vi "LocalQueue_Test No Connection Errors.vi"(8 "error in (no error)":errorcluster) -> (0 "error out":errorcluster)   [LabVIEW 2013]
uses:
  <vilib>/addons/_JKI Toolkits/Caraya/classes/Assert/Assert Equal Value_Variant.vi
  <vilib>/LabVIEW Open Source Project/Connection/Connection/Connection.lvclass
  <vilib>/addons/_JKI Toolkits/Caraya/classes/Test/Test.lvclass
  <vilib>/addons/_JKI Toolkits/Caraya/classes/Assert/Assert.lvclass
  source/MQTT_LocalQueue/Connection/LocalQueueConnection.lvclass
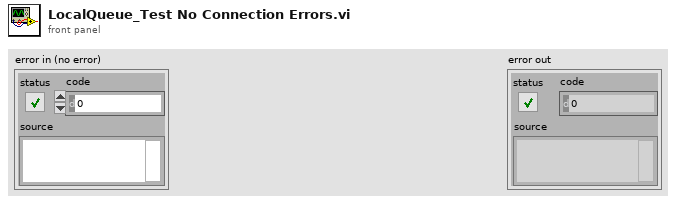
[diagram p1: front panel]
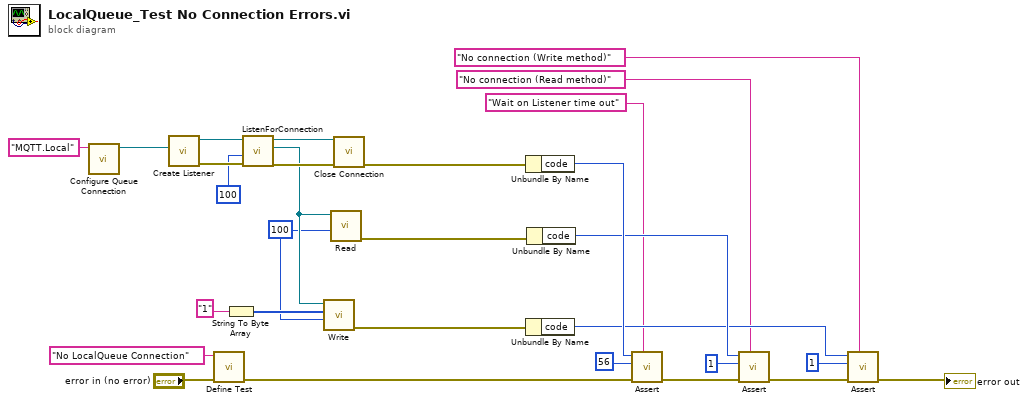
[diagram p0: block diagram]
diagram:
  w3 = 100 ("bytes to read")
  n1 = call "Configure Queue Connection.vi"("Queue Name"="MQTT.Local") -> ("LocalQueueConnection"=w2:refnum<class "LocalQueueConnection.lvclass">)  [unwired: 9 in, 1 out]
  n2 = call <vilib>:"Create Listener.vi"("Connection Configuration"=w2) -> ("error out"=w26:errorcluster, "Listener"=w29:refnum<class "LocalQueueConnection.lvclass">)  [unwired: 9 in]
  n3 = call <vilib>:"Define Test.vi"("error in (no error)"="error in (no error)", "Label (VI Title)"="No LocalQueue Connection") -> ("error out"=w17:errorcluster)  [unwired: 9 in]
  n4 = String To Byte Array(string="1" ("data in")) -> (unsigned byte array=w24:u8[])
  n5 = call <vilib>:"ListenForConnection.vi"("error in (no error)"=w26, "timeout (2000 ms)"=100 ("timeout ms (wait forever: -1)"), "Listener"=w29) -> ("error out"=w27:errorcluster, "Connection"=w22:refnum<class "Connection.lvclass">, "Listener out"=w28:refnum<class "LocalQueueConnection.lvclass">)  [unwired: 5 in, 1 out]
  n6 = call <vilib>:"Write.vi"("timeout (2000 ms)"=w3, "Bytes"=w24, "Connection in"=w22) -> ("error out"=w20:errorcluster)  [unwired: 7 in, 1 out]
  n7 = call <vilib>:"Read.vi"("timeout (2000 ms)"=w3, "TCPConnection in"=w22) -> ("error out"=w19:errorcluster)  [unwired: 5 in, 4 out]
  n8 = call <vilib>:"Close Connection.vi"("error in (no error)"=w27, "Connection in"=w28) -> ("error out"=w21:errorcluster)  [unwired: 8 in, 1 out]
  n9 = Unbundle By Name(w21) -> ("code"=w16:i32)
  n10 = Unbundle By Name(w20) -> ("code"=w11:i32)
  n11 = Unbundle By Name(w19) -> ("code"=w12:i32)
  n12 = call-poly <vilib>:"Assert.vi"("Label"="Wait on Listener time out" ("Label (VI Title)"), "error in (no error)"=w17, "Y"=56 ("code"), "X"=w16) -> ("error out"=w14:errorcluster)  [unwired: 7 in]
  n13 = call-poly <vilib>:"Assert.vi"("Label"="No connection (Read method)" ("Label (VI Title)"), "error in (no error)"=w14, "Y"=1 ("code"), "X"=w12) -> ("error out"=w13:errorcluster)  [unwired: 7 in]
  n14 = call-poly <vilib>:"Assert.vi"("Label"="No connection (Write method)" ("Label (VI Title)"), "error in (no error)"=w13, "Y"=1 ("code"), "X"=w11) -> ("error out"=→"error out":errorcluster)  [unwired: 7 in]
